vi "Set_Items.vi"   [LabVIEW 2020, in "CtlReferences.lvlib" / "CtlReferences.lvclass"]
uses:
  CtlReferences.lvclass
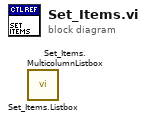
[diagram p0: block diagram]
diagram:
  n1 = call "Set_Items.Listbox.vi"() -> ()  [unwired: 9 in, 3 out]
  n2 = call "Set_Items.MulticolumnListbox.vi"() -> ()  [unwired: 9 in, 3 out]
